vi "AinContinuous.vi"() -> ()   [LabVIEW 2010]
uses:
  <userlib>/LV-LINK/PolySubVIs/CreateAinChan.vi
  <userlib>/LV-LINK/PolySubVIs/OLTimingSetInput.vi
  <userlib>/LV-LINK/PolySubVIs/OLReadMultiple2D.vi
panel:
  out "Waveform Chart":dbl[][](graph)
  out "Acquired Data":dbl[][](graph)
  in  "Samples Per Channel":dbl=1000.0
  in  "Sample Rate":dbl=10000.0
  in  "?":bool
  in  "Channels":string="Ain 0"
  # "Continuous Analog Input Example"
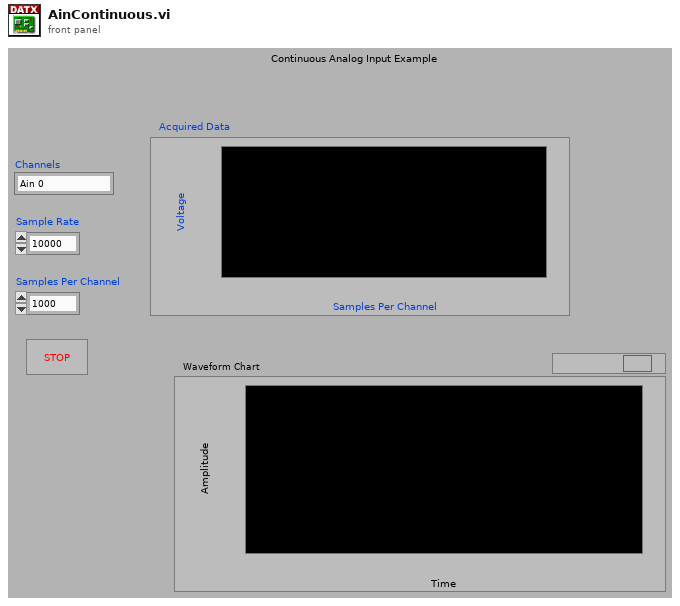
[diagram p1: front panel]
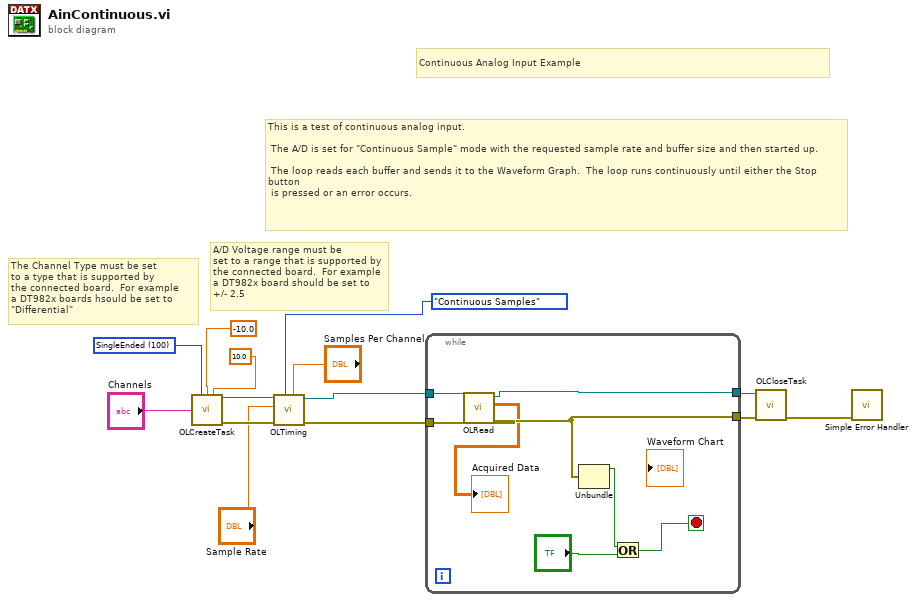
[diagram p0: block diagram]
diagram:
  w4 = 100 items=["SingleEnded"=100, "Differential"=101] ("Channel Type")
  # "The Channel Type must be set\nto a type that is supported by \nthe connected board.  For example\na DT982x boards hsould be set to\n\"Differential\""
  # "A/D Voltage range must be\nset to a range that is supported by \nthe connected board.  For example\na DT982x board should be set to \n+/- 2.5"
  # "Continuous Analog Input Example"
  # "This is a test of continuous analog input. \n\n The A/D is set for \"Continuous Sample\" mode with the requested sample rate and buffer size and then started up.\n\n The loop reads each buffer and sends it to the Waveform Graph.  The loop runs continuously until either the Stop button\n is pressed or an error occurs."
  n1 = call-poly <userlib>:"OLCreateTask.vi"("Channel Type"=w4, "Range Min"=-10.0, "Range Max"=10.0, "Channel"="Channels") -> ("Task Out"=w2:refnum<k24>, "error out"=w13:errorcluster)  [unwired: 10 in]
  n2 = call-poly <userlib>:"OLTiming.vi"("Samples Per Channel"="Samples Per Channel", "Sample Mode"=enum16{"Finite Samples", "Continuous Samples"}."Continuous Samples", "error in (no error)"=w13, "Sample Freq (Hz)"="Sample Rate", "Task In"=w2) -> ("error out"=w5:errorcluster, "Task Out"=w6:refnum<k24>)  [unwired: 4 in, 1 out]
  n3 = while {
    tunnel: w5 -> [w22]
    tunnel: [w21] -> w8
    tunnel: [w20] -> w7
    tunnel: w6 -> [w17]
    stop <- w16 stop-if-true
    n4 = call-poly <userlib>:"OLRead.vi"("error in (no error)"=w22, "Task In"=w17) -> ("error out"=w20:errorcluster, "ReadData"=→"Acquired Data":dbl[][], "Task Out"=w21:refnum<k24>)  [unwired: 7 in]
    n5 = Unbundle(w20) -> ("status"=w19:bool)  [unwired: 2 out]
    n6 = Or(x=w19, y="?") -> (x .or. y?=w16:bool)
  }
  n7 = call <userlib>:"OLCloseTask.vi"("Error in"=w7, "Task In"=w8) -> ("Error Out"=w10:errorcluster)  [unwired: 9 in]
  n8 = call <vilib>:"Simple Error Handler.vi"("error in (no error)"=w10) -> ()  [unwired: 4 in, 5 out]
